vi "Initialize.vi"(8 "error in":errorcluster, 10 "Plugin Name":string, 11 "Voltage Control in":refnum<class "Voltage Control.lvclass">) -> (0 "error out":errorcluster, 3 "Voltage Control out":refnum<class "Voltage Control.lvclass">)   [LabVIEW 2023, in "Voltage Control.lvclass"]
uses:
  Voltage Control.lvclass
  Voltage Control.lvclass/Voltage Control.ctl
  <vilib>/ADAS Replay HIL/Channels/Tag Wrapper/Polymorphic/Open Consumer Tag (Double).vi
  <vilib>/ADAS Replay HIL/Channels/Tag Wrapper/Polymorphic/Open Consumer Tag (Double).vi/bacb721e-673a-491a-accd-959f2e1f334e.vi
  <vilib>/ADAS Replay HIL/Channels/Tag Wrapper/Polymorphic/Open Consumer Tag (Double).vi/bacb721e-673a-491a-accd-959f2e1f334e.vi/c28b0ead-42ad-4072-80a2-aca7f2bd7ce3.vi
  <vilib>/ADAS Replay HIL/AdasHilServices/AdasHilServices Fill In Error Info Ex.vi
  <vilib>/ADAS Replay HIL/Channels/Tag Wrapper/Tag Wrapper.lvlib
  Capability/Capability.lvclass
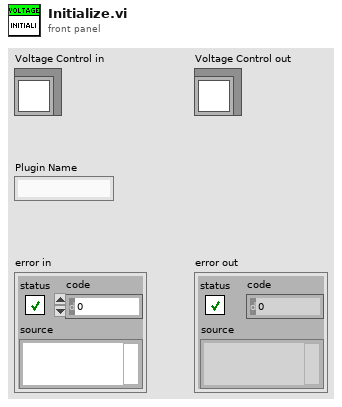
[diagram p1: front panel]
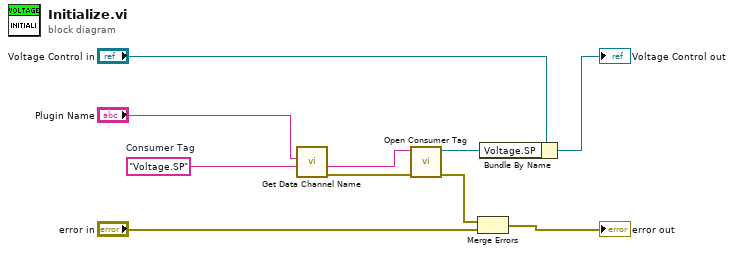
[diagram p0: block diagram]
diagram:
  w10 = "Voltage.SP"  # Consumer Tag
  n1 = call "Get Data Channel Name.vi"("Channel Name"=w10, "Plugin Name"="Plugin Name") -> ("error out"=w7:errorcluster, "Data Channel Name"=w9:string)  [unwired: 8 in]
  n2 = call-poly <vilib>:"Open Consumer Tag.vi"("error in"=w7, "Channel Name"=w9) -> ("error out"=w4:errorcluster, "ADAS HIL Channel"=w1:refnum<k21>)  [unwired: 8 in]
  n3 = Merge Errors(w4, "error in") -> (→"error out":errorcluster)
  n4 = Bundle By Name(cluster="Voltage Control in", "Voltage.SP"=w1) -> (→"Voltage Control out":refnum<class "Voltage Control.lvclass">)
